vi "first state selector.vi"(8 "error in":errorcluster, 10 "state":T2=enum."Low pressure", 11 "Simulation Controls":T1) -> (0 "error out":errorcluster, 3 "state out":T2)   [LabVIEW 2015]
uses:
  controls/state.ctl
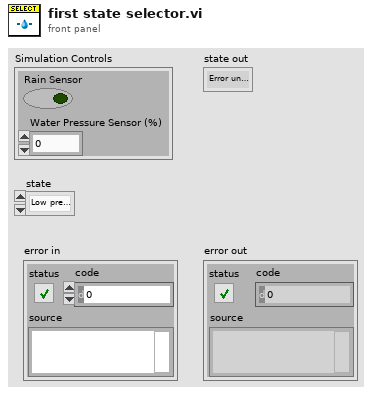
[diagram p1: front panel]
types:
  T1 = cluster{"Rain Sensor":bool, "Water Pressure Sensor (%)":dbl}
  T2 = typedef "state.ctl" = enum16{"Error under range", "Exit", "Initialize", "Start", "Error", "Run", "Setup", "Low pressure", "Rain", "Idle"}
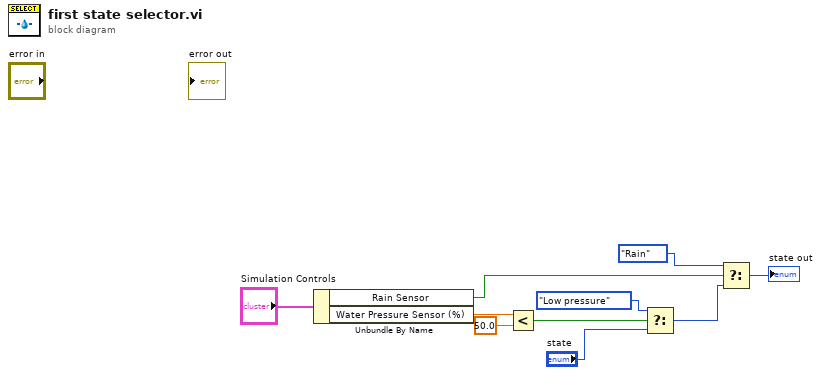
[diagram p0: block diagram]
diagram:
  n1 = Unbundle By Name("Simulation Controls") -> ("Rain Sensor"=w7:bool, "Water Pressure Sensor (%)"=w2:dbl)
  n2 = Less?(x=w2, y=50.0) -> (x < y?=w4:bool)
  n3 = Select(t=state."Low pressure" ("state"), s=w4, f="state") -> (s? t:f=w9:T2)
  n4 = Select(t=state."Rain" ("state"), s=w7, f=w9) -> (s? t:f=→"state out":T2)
